vi "Read_Sonar.vi"(0 "error in":errorcluster, 3 "node":string) -> (1 "error out":errorcluster, 4 "Point Cloud":T1)   [LabVIEW 2012]
doc: "This VI returns point cloud from the head sonar readings"
uses:
  <userlib>/ROS for LabVIEW Software/ROS/Code/Console/Servers/ServerSubs/TopicDef.ctl
  <userlib>/ROS for LabVIEW Software/ROS/Code/SubVIs/_ROSDirection.ctl
panel:
  out "Reply":string
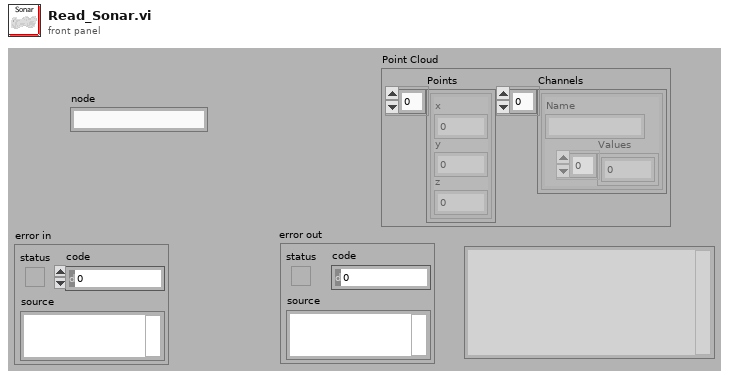
[diagram p1: front panel]
types:
  T1 = cluster{"Points":cluster{"x":sgl, "y":sgl, "z":sgl}[], "Channels":cluster{"Name":string, "Values":sgl[]}[]}
  T2 = typedef "TopicDef.ctl" = cluster{"Topic":string, "Type":string, "Action":T3, "Update (ms)":u16, "queue size":u16}
  T3 = typedef "_ROSDirection.ctl" = enum16{"Node", "Publisher", "Subscriber", "ServiceClient", "ServiceProvider"}
  T4 = typedef "_ROSControl.ctl" = cluster{"topic port":u16, "Node":string, "topic":string, "type":string, "node port":u16, "error ":errorcluster, "Direction":T3, "Update (ms)":u16, "FIFO size":u16}
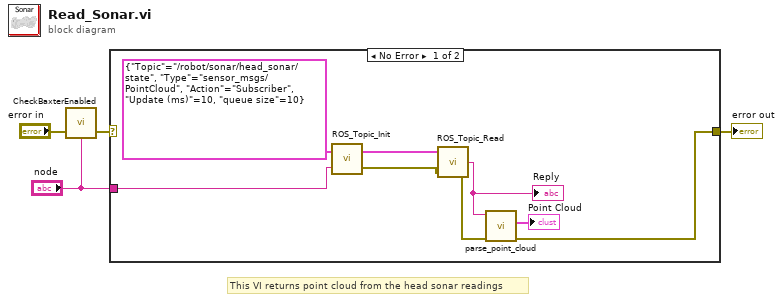
[diagram p0: block diagram]
diagram:
  # "This VI returns point cloud from the head sonar readings"
  n1 = call <userlib>:"CheckBaxterEnabled.vi"("error in"="error in", "node"="node") -> ("error out"=w2:errorcluster)  [unwired: 2 in]
  n2 = case shown="No Error" w2 {
    selector: w2 -> [_ w13]
    tunnel: [w5 w13] -> w4
    tunnel: "node" -> [w8 _]
    frame No Error {
      n3 = call <userlib>:"ROS_Topic_Init.vi"("node"=w8, "Definitions"=T2 {"Topic"="/robot/sonar/head_sonar/state", "Type"="sensor_msgs/PointCloud", "Action"=enum."Subscriber", "Update (ms)"=10, "queue size"=10}) -> ("error out"=w7:errorcluster, "ROS out"=w12:T4)
      n4 = call <userlib>:"ROS_Topic_Read.vi"("error in (no error)"=w7, "ROS in"=w12) -> ("error out"=w6:errorcluster, "Reply"=w11:string)  [unwired: 1 in, 1 out]
      "Reply" <- w11
      n5 = call <userlib>:"parse_point_cloud.vi"("error in"=w6, "msg in"=w11) -> ("error out"=w5:errorcluster, "Point Cloud"=→"Point Cloud":T1)  [unwired: 2 in, 2 out]
    }
    frame Error {
    }
  }
  "error out" <- w4
